vi "CAN ISA Write.vi"(0 "ID":u32, 1 "MSG type":T1(ring), 2 "LEN":u8, 3 "Data":u8[](array[numeric])) -> (5 "Error Number":u32 format="%.0x")   [LabVIEW 2009]
doc: "CAN Write schreibt eine Nachricht in die Sende-Queue des Treibers. Rückgabe ist ein Fehlercode wie er in den Header-Dateien beschrieben ist."
uses:
  PCAN_ISA.dll
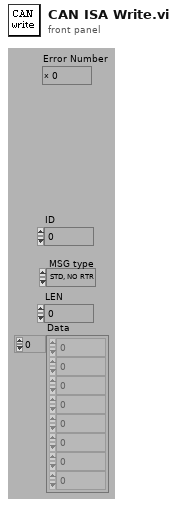
[diagram p1: front panel]
types:
  T1 = enum8{"STD, NO RTR", "STD,RTR", "XTD, NO RTR", "XTD, RTR"}
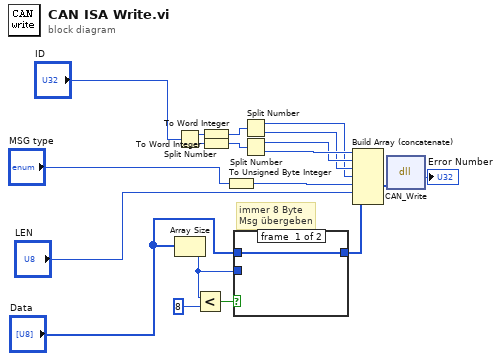
[diagram p0: block diagram]
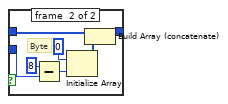
[diagram p2: hidden frame]
diagram:
  # "immer 8 Byte\nMsg übergeben"
  n1 = Split Number(x="ID") -> (hi(x)=w11:u16, lo(x)=w12:u16)
  n2 = Array Size(array="Data") -> (size(s)=w8:i32)
  n3 = Less?(x=w8, y=8) -> (x < y?=w7:bool)
  n4 = To Word Integer(number=w11) -> (16bit integer=w14:i16)
  n5 = To Word Integer(number=w12) -> (16bit integer=w15:i16)
  n6 = To Unsigned Byte Integer(number="MSG type") -> (unsigned 8bit integer=w13:u8)
  n7 = case shown="True" w7 {
    tunnel: "Data" -> [w20 w23]
    tunnel: [w20 w22] -> w5
    tunnel: w8 -> [_ w27]
    frame #0 {
    }
    frame #1 {
      # "Byte"
      n8 = Subtract(x=8, y=w27) -> (x-y=w25:i32)
      n9 = Initialize Array(i8 0, w25) -> (w21:i8[])
      n10 = Build Array (concatenate)(w23, w21) -> (w22:u8[])
    }
  }
  n11 = Split Number(x=w14) -> (hi(x)=w16:u8, lo(x)=w17:u8)
  n12 = Split Number(x=w15) -> (hi(x)=w18:u8, lo(x)=w19:u8)
  n13 = Build Array (concatenate)(w19, w18, w17, w16, w13, "LEN", w5) -> (w10:u8[])
  n14 = dll-call lib="C:/Documents and Settings/PQ/Desktop/LabView-Dateien/PCAN_ISA.dll" fn="CAN_Write"("TPCANMsg"=w10) -> ("Error Number"=→"Error Number":u32)  [unwired: 4 in, 2 out]
